vi "Connect Trigger Terminals-Array.vi"(8 "error in (no error)":errorcluster, 10 "Routing Information":T1[](array[typedef]), 11 "instrument handle":refnum<k15>) -> (0 "error out":errorcluster, 3 "instrument handle out":refnum<k15>)   [LabVIEW 2026]
doc: "This VI allows an array input of Trigger Routing Controls. NI-SYNC will make the connects of each array input. The benefit of this vi is there is no need for multiple string inputs."
uses:
  Trigger Routing.ctl
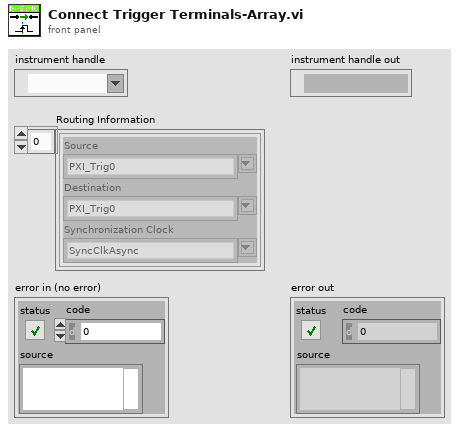
[diagram p1: front panel]
types:
  T1 = typedef "Trigger Routing.ctl" = cluster{"Source":string, "Destination":string, "Synchronization Clock":string}
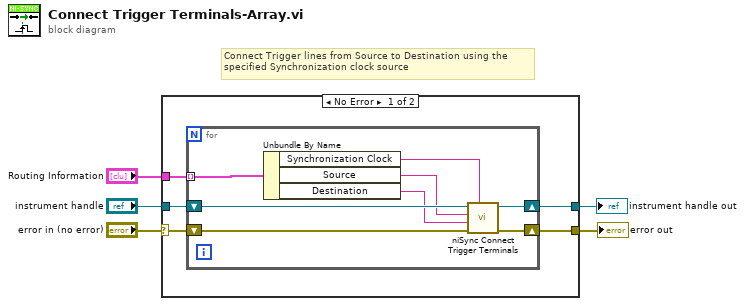
[diagram p0: block diagram]
diagram:
  # "Connect Trigger lines from Source to Destination using the\nspecified Synchronization clock source"
  n1 = case shown="No Error" "error in (no error)" {
    selector: "error in (no error)" -> [w7 w20]
    tunnel: "Routing Information" -> [w10 _]
    tunnel: "instrument handle" -> [w9 w19]
    tunnel: [w8 w19] -> w4
    tunnel: [w6 w20] -> w2
    frame No Error {
      n2 = for {
        tunnel: w10 -> [w18] mode=indexing
        shift-right: [w16] -> w8
        shift-left: w9 -> [w17]
        shift-right: [w14] -> w6
        shift-left: w7 -> [w15]
        n3 = Unbundle By Name(w18) -> ("Synchronization Clock"=w13:string, "Source"=w12:string, "Destination"=w11:string)
        n4 = call <instrlib>:"niSync Connect Trigger Terminals.vi"("synchronization clock"=w13, "error in (no error)"=w15, "destination terminal"=w11, "source terminal"=w12, "instrument handle"=w17) -> ("error out"=w14:errorcluster, "instrument handle out"=w16:refnum<k15>)  [unwired: 5 in]
      }
    }
    frame Error {
    }
  }
  "instrument handle out" <- w4
  "error out" <- w2
